vi "App_Main.vi"() -> ()   [LabVIEW 2012]
uses:
  SupportVi/LineStateLamp.ctl
  Fun/Dev/SupportVi/DevState.ctl
  Fun/Dev/DevControl.lvclass
  SupportVi/SystemState.ctl
  Fun/Http/HttpClient.lvclass
  SupportVi/Dev_State_Color.ctl
  <vilib>/Utility/miscctls.llb/LVRowAndColumnTypeDef.ctl
  Fun/Dev/SupportVi/LampState.ctl
  Libs/Ini/ProcessMode.ctl
  <vilib>/Utility/miscctls.llb/LVRowAndColumnUnsignedTypeDef.ctl
  Libs/Ini/IniReader&WriterForControl.lvlib
panel:
  out "Fac&FloChkOK?":bool
  out "HttpClient":refnum<class "HttpClient.lvclass">
  out "FloorCode":string
  out "FactoryCode":string
  out "有變化的部分":string
  in  "Ïµ½y î‘B":T1=enum."Quit"
  out "ˆó¾¯Æ÷":refnum<class "DevControl.lvclass">
  out "需要掃描的":T3(array[cluster])
  out "所有的":cluster{"Addr":u8, "Enable?":bool}[](array[cluster])
  out "History":path
  out "Port":refnum<visa-resource-name>
  out "ConfigFile":path
  out "DataUpload":bool
  out "ReadDelay":i32
  out "SerialRetry":i32
  out "LampBaudRate":i32
  out "BaudRate":i32
  in  "VerifyTimes":i32
  out "DataUrl":string
  out "Model":string
  out "Line":string
  out "Floor":string
  out "Factory":string
  out "RootPath":path
  in  "運行信息":string
  out "版本信息":string
  out "LineState":T4
  out "No-Reply":u32(colorbox)
  out "Abnormal":u32(colorbox)
  in  "ESDShower":string[][](table)
  out "Normal":u32(colorbox)
  in  "Stop":bool
  in  "Start":bool
  # "ESD Monitor System"
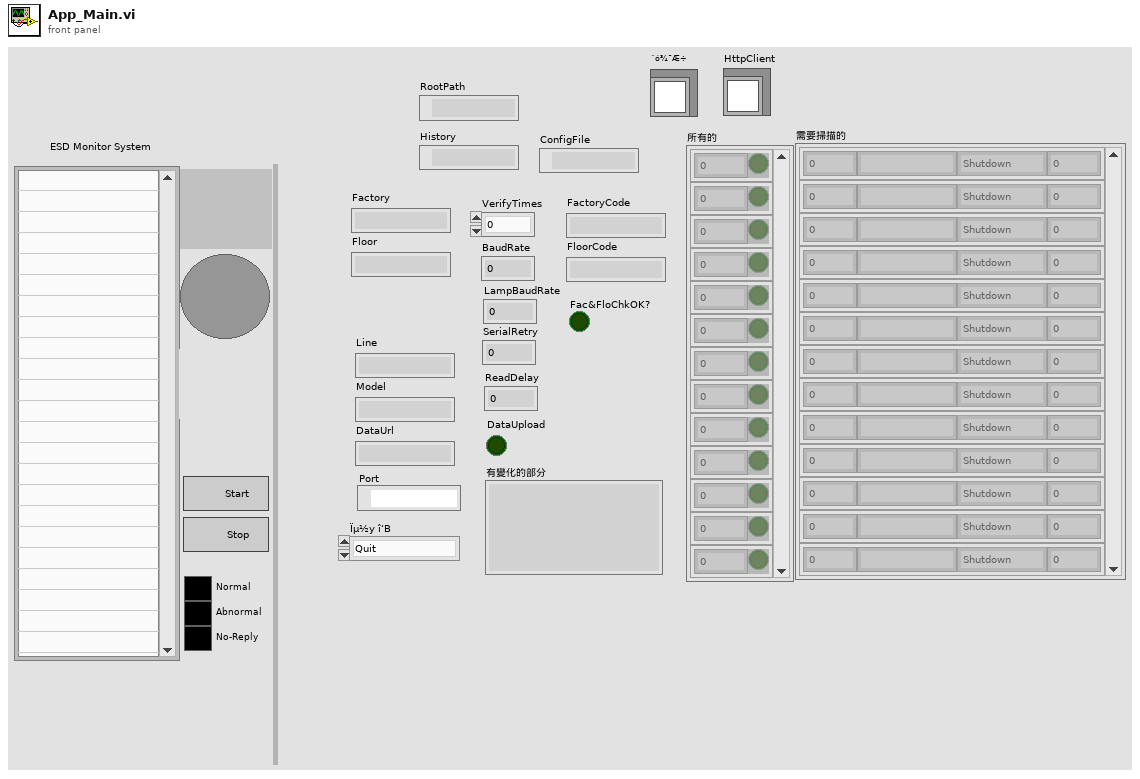
[diagram p1: front panel]
types:
  T1 = typedef "SystemState.ctl" = enum16{"Pause", "Quit", "Error", "Stopping", "Starting", "Init", "Scan", "Menu", "ReadConf", "Idle"}
  T2 = typedef "DevControl.lvclass/DevState.ctl" = enum16{"Shutdown", "PASS", "FAIL", "Idle", "Noresponse"}
  T3 = cluster{"Addr":u8, "name":string, "State":T2, "Retry":i32}[]
  T4 = typedef "LineStateLamp.ctl" = bool
  T5 = typedef "Dev_State_Color.ctl" = u32
  T6 = typedef "IniReader&WriterForControl.lvlib/ProcessMode.ctl" = enum16{"读", "写"}
  T7 = enum8{"Enabled", "Disabled", "Disabled and Grayed Out"}
  T8 = typedef "LVRowAndColumnUnsignedTypeDef.ctl" = cluster{"Row":u32, "Column":u32}
  T9 = cluster{"Addr":i32, "name":string, "State":T2, "Retry":i32}[]
  T10 = typedef "LVRowAndColumnTypeDef.ctl" = cluster{"Row":i32, "Column":i32}
  T11 = typedef "DevControl.lvclass/LampState.ctl" = enum16{"üS+·äøQÆ÷", "¼t+·äøQÆ÷", "·äøQÆ÷", "È«œç", "全亮", "üS", "¾G", "¼t"}
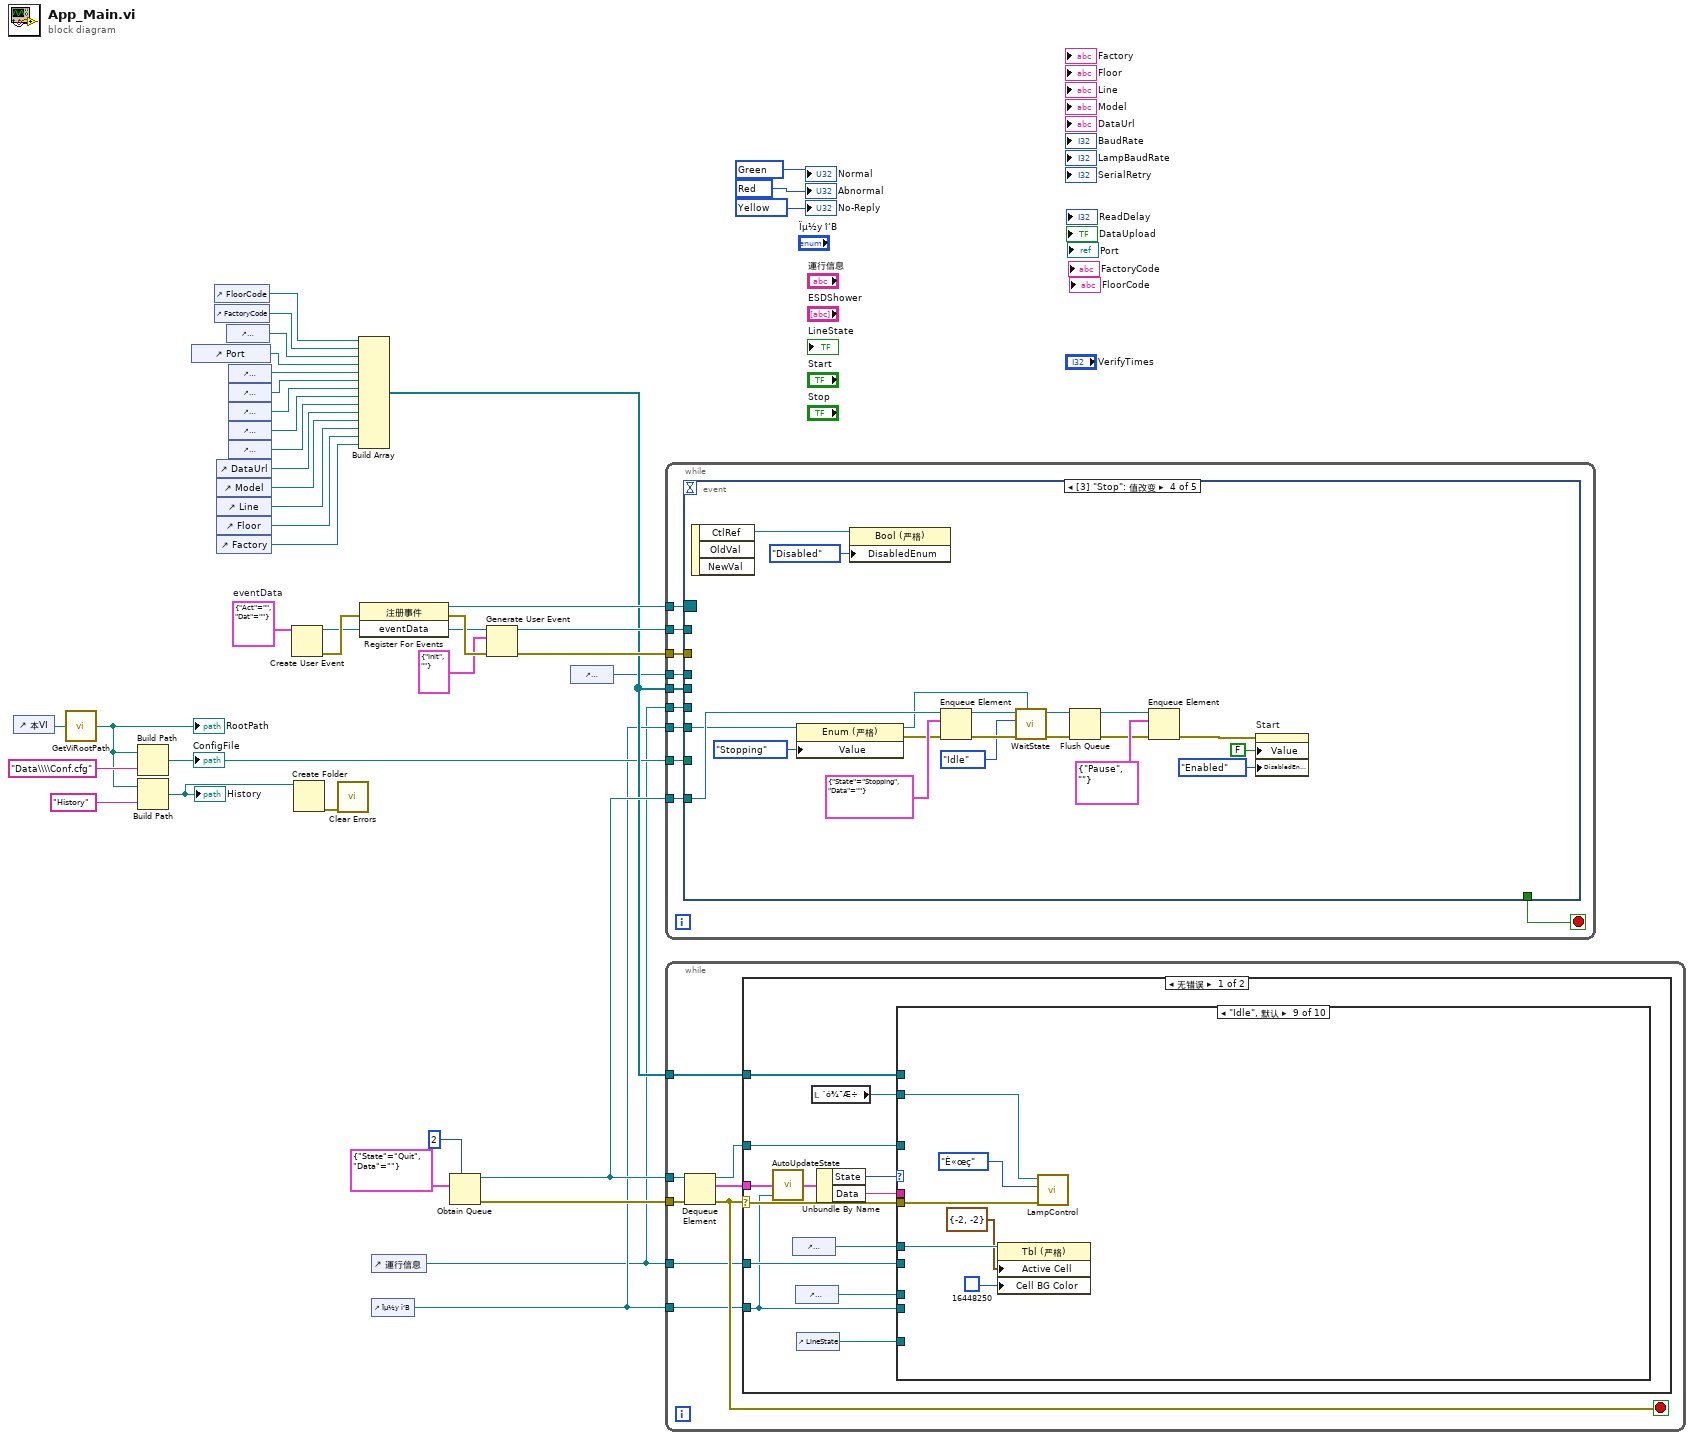
[diagram p0: block diagram]
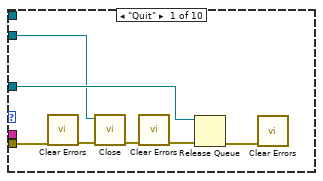
[diagram p2: hidden frame]
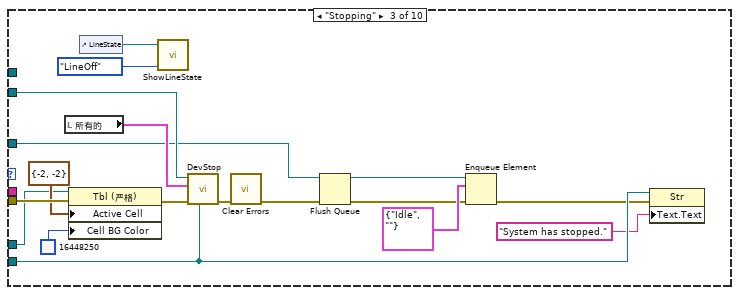
[diagram p4: hidden frame]
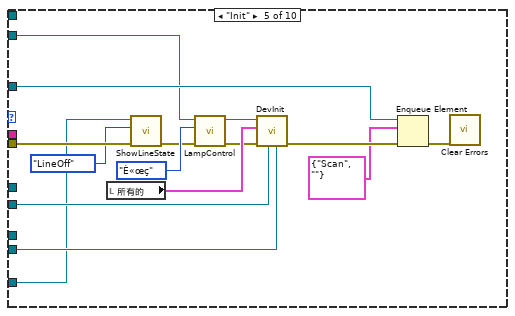
[diagram p6: hidden frame]
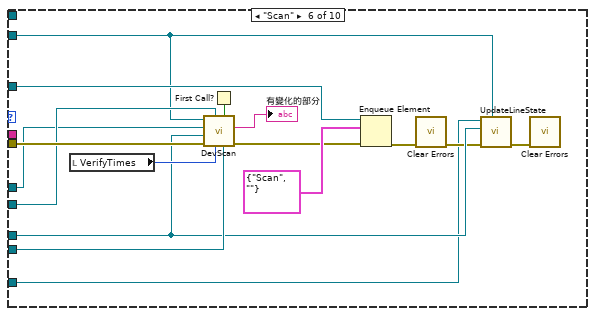
[diagram p7: hidden frame]
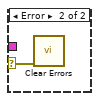
[diagram p11: hidden frame]
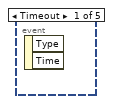
[diagram p12: hidden frame]
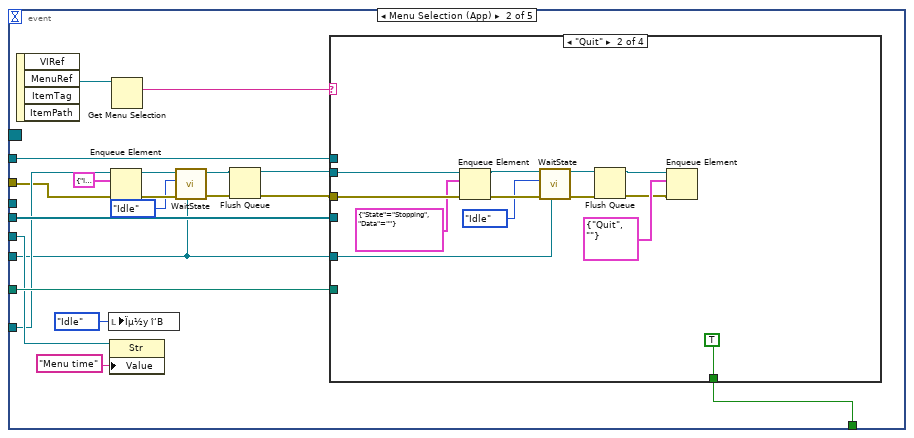
[diagram p13: hidden frame]
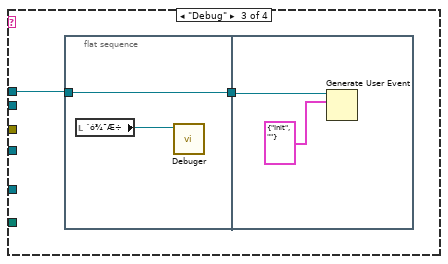
[diagram p15: hidden frame]
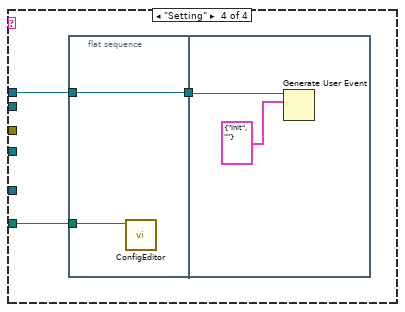
[diagram p16: hidden frame]
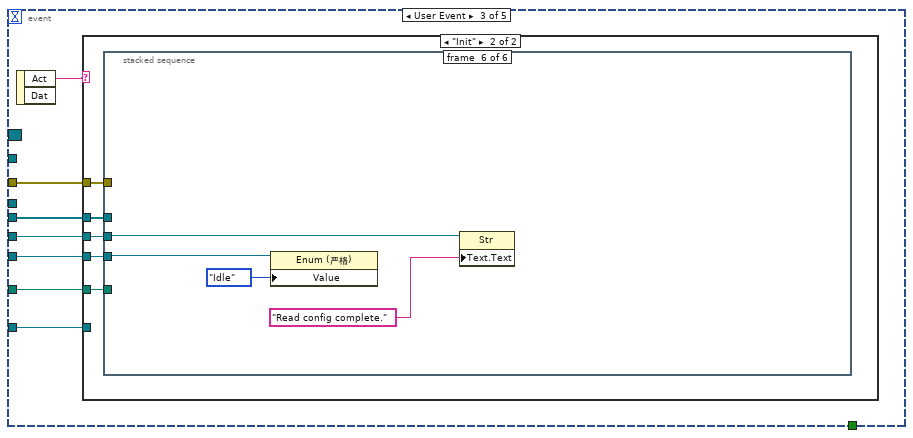
[diagram p17: hidden frame]
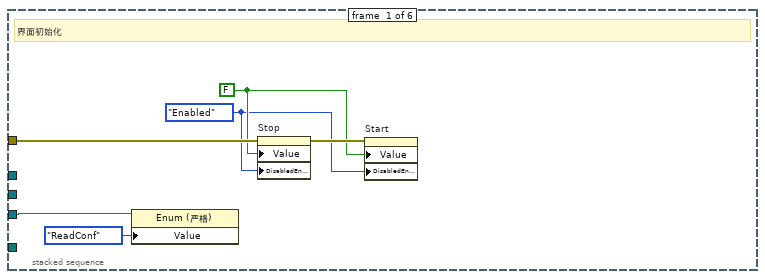
[diagram p19: hidden frame]
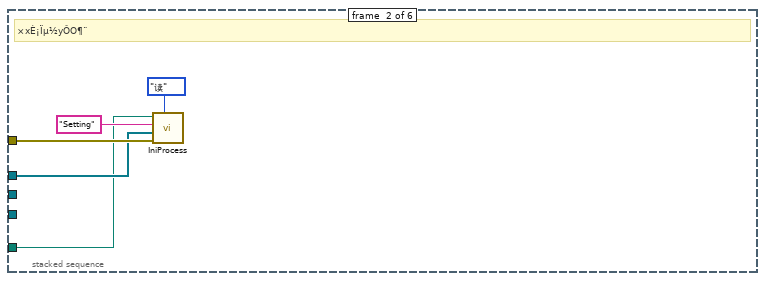
[diagram p20: hidden frame]
diagram:
  w32 = cluster{"Act":string, "Dat":string} {"Act"="", "Dat"=""}  # eventData
  w38 = T5 16772209 items=["Yellow"=16772209, "Red"=16711680, "Green"=6618880] ("DevState_Color")
  w39 = T5 16711680 items=["Yellow"=16772209, "Red"=16711680, "Green"=6618880] ("DevState_Color")
  w40 = T5 6618880 items=["Yellow"=16772209, "Red"=16711680, "Green"=6618880] ("DevState_Color")
  n1 = control-ref of="本VI"() -> (w37:refnum<vi>)
  n2 = call "GetViRootPath.vi"("VI引用句柄"=w37) -> ("RootPath"=w12:path)
  "RootPath" <- w12
  n3 = Build Path(base path=w12, name or relative path="Data\\\\Conf.cfg" ("名称或相对路径")) -> (appended path=w7:path)
  "ConfigFile" <- w7
  n4 = Build Path(base path=w12, name or relative path="History" ("名称或相对路径")) -> (appended path=w10:path)
  "History" <- w10
  n5 = control-ref of="Port"() -> (w14:refnum<vi>)
  n6 = control-ref of="FloorCode"() -> (w2:refnum<vi>)
  n7 = control-ref of="FactoryCode"() -> (w3:refnum<vi>)
  n8 = control-ref of="DataUrl"() -> (w20:refnum<vi>)
  n9 = control-ref of="Model"() -> (w19:refnum<vi>)
  n10 = control-ref of="Line"() -> (w18:refnum<vi>)
  n11 = control-ref of="Floor"() -> (w17:refnum<vi>)
  n12 = control-ref of="Factory"() -> (w16:refnum<vi>)
  n13 = control-ref of="VerifyTimes"() -> (w13:refnum<vi>)
  n14 = control-ref of="DataUpload"() -> (w25:refnum<vi>)
  n15 = control-ref of="ReadDelay"() -> (w24:refnum<vi>)
  n16 = control-ref of="SerialRetry"() -> (w23:refnum<vi>)
  n17 = control-ref of="LampBaudRate"() -> (w22:refnum<vi>)
  n18 = control-ref of="BaudRate"() -> (w21:refnum<vi>)
  n19 = Create User Event(user event datatype=w32) -> (user event=w29:refnum<user-event>, error out=w31:errorcluster)  [unwired: 1 in]
  n20 = Create Folder(path (use dialog)=w10) -> (error out=w8:errorcluster)  [unwired: 2 in, 2 out]
  n21 = call <vilib>:"Clear Errors.vi"("error in (no error)"=w8) -> ()  [unwired: 6 in, 1 out]
  n22 = Build Array(w2, w3, w13, w14, w25, w24, w23, w22, w21, w20, w19, w18, w17, w16) -> (w9:refnum<vi>[])
  n23 = register-events(error in=w31, w29) -> (reference out=w33:refnum<event-registration>, error out=w30:errorcluster)  [unwired: 1 in]
  n24 = control-ref of="運行信息"() -> (w5:refnum<vi>)
  n25 = control-ref of="Ïµ½y î‘B"() -> (w6:refnum<vi>)
  n26 = Obtain Queue(max queue size (-1, unlimited)=2 ("队列最大值（-1，无限）"), element data type=cluster{"State":T1, "Data":string} {"State"=enum."Quit", "Data"=""}) -> (queue out=w34:refnum<queue>, error out=w36:errorcluster)  [unwired: 3 in, 1 out]
  n27 = Generate User Event(user event=w29, event data cluster=cluster{"Act":string, "Dat":string} {"Act"="Init", "Dat"=""} ("事件数据"), error in=w30) -> (user event out=w27:refnum<user-event>, error out=w26:errorcluster)
  n28 = control-ref of="ESDShower"() -> (w4:refnum<vi>)
  n29 = while {
    tunnel: w34 -> [w49]
    tunnel: w33 -> [w48]
    tunnel: w27 -> [w47]
    tunnel: w26 -> [w46]
    tunnel: w9 -> [w45]
    tunnel: w7 -> [w44]
    tunnel: w6 -> [w43]
    tunnel: w5 -> [w42]
    tunnel: w4 -> [w41]
    stop <- w50 stop-if-true
    n30 = event shown="[3] \"Stop\": 值改变" {
      selector: w48 -> [_ _ _ _ _]
      dyn-events: _ -> [_ _ _ _ _]
      timeout: _ -> [_ _ _ _ _]
      tunnel: [_ w67 _ _ w191] -> w50
      tunnel: w49 -> [_ w60 w100 w180 w192]
      tunnel: w47 -> [_ w63 _ _ _]
      tunnel: w46 -> [_ w59 w99 _ w184]
      tunnel: w45 -> [_ w65 w98 _ _]
      tunnel: w44 -> [_ w64 w97 _ _]
      tunnel: w43 -> [_ w57 w96 w178 _]
      tunnel: w42 -> [_ w62 w95 _ _]
      tunnel: w41 -> [_ _ _ _ w188]
      event Timeout {
        n31 = event-data() -> ()  [unwired: 1 in, 2 out]
      }
      event Menu Selection (App) {
        n32 = event-data() -> ("MenuRef"=w69:refnum<k9>)  [unwired: 1 in, 3 out]
        n33 = local write "Ïµ½y î‘B"(SystemState."Idle" ("Ïµ½y î‘B")) -> ()
        n34 = property class="Str"(reference=w62, "Value"="Menu time" ("值")) -> ()  [unwired: 1 in, 2 out]
        n35 = Enqueue Element(queue=w60, element=cluster{"State":T1, "Data":string} {"State"=enum."Idle", "Data"=""} ("元素"), error in (no error)=w59) -> (queue out=w53:refnum<queue>, error out=w58:errorcluster)  [unwired: 1 in, 1 out]
        n36 = Get Menu Selection(0:w69) -> (6:w68:string)  [unwired: 3 in, 4 out]
        n37 = call "WaitState.vi"("Enum输入"=w57, "错误输入（无错误）"=w58, "™z²é î‘B"=SystemState."Idle") -> ("错误输出"=w55:errorcluster)  [unwired: 8 in]
        n38 = Flush Queue(queue=w53, error in (no error)=w55) -> (queue out=w52:refnum<queue>, error out=w54:errorcluster)  [unwired: 1 out]
        n39 = case shown="\"Quit\"" w68 {
          tunnel: [_ TRUE _ _] -> w67
          tunnel: w54 -> [_ w78 _ _]
          tunnel: w65 -> [_ _ _ _]
          tunnel: w64 -> [_ _ _ w90]
          tunnel: w52 -> [_ w79 _ _]
          tunnel: w63 -> [_ _ w82 w89]
          tunnel: w57 -> [_ w75 _ _]
          frame "假", Default {
          }
          frame "Quit" {
            n40 = Enqueue Element(queue=w79, element=cluster{"State":T1, "Data":string} {"State"=enum."Stopping", "Data"=""} ("元素"), error in (no error)=w78) -> (queue out=w72:refnum<queue>, error out=w76:errorcluster)  [unwired: 1 in, 1 out]
            n41 = call "WaitState.vi"("Enum输入"=w75, "错误输入（无错误）"=w76, "™z²é î‘B"=SystemState."Idle") -> ("错误输出"=w73:errorcluster)  [unwired: 8 in]
            n42 = Flush Queue(queue=w72, error in (no error)=w73) -> (queue out=w70:refnum<queue>, error out=w71:errorcluster)  [unwired: 1 out]
            n43 = Enqueue Element(queue=w70, element=cluster{"State":T1, "Data":string} {"State"=enum."Quit", "Data"=""} ("元素"), error in (no error)=w71) -> ()  [unwired: 1 in, 3 out]
          }
          frame "Debug" {
            n44 = flat-sequence {
              tunnel: w82 -> [w85]
              tunnel: [w85] -> w83
              tunnel: w83 -> [w87]
              frame #0 {
                n45 = local read "ˆó¾¯Æ÷"() -> (w84:refnum<class "DevControl.lvclass">)
                n46 = call "Debuger.vi"("DevControl输入"=w84) -> ()  [unwired: 11 in]
              }
              frame #1 {
                n47 = Generate User Event(user event=w87, event data cluster=cluster{"Act":string, "Dat":string} {"Act"="Init", "Dat"=""} ("事件数据")) -> ()  [unwired: 1 in, 2 out]
              }
            }
          }
          frame "Setting" {
            n48 = flat-sequence {
              tunnel: w90 -> [w92]
              tunnel: w89 -> [w91]
              tunnel: [w91] -> w88
              tunnel: w88 -> [w94]
              frame #0 {
                n49 = call "ConfigEditor.vi"("ConfigFile"=w92) -> ()  [unwired: 11 in]
              }
              frame #1 {
                n50 = Generate User Event(user event=w94, event data cluster=cluster{"Act":string, "Dat":string} {"Act"="Init", "Dat"=""} ("事件数据")) -> ()  [unwired: 1 in, 2 out]
              }
            }
          }
        }
      }
      event User Event {
        n51 = event-data() -> ("Act"=w101:string)  [unwired: 1 in, 1 out]
        n52 = case shown="\"Init\"" w101 {
          tunnel: w100 -> [_ _]
          tunnel: w99 -> [_ w106]
          tunnel: w98 -> [_ w105]
          tunnel: w97 -> [_ w104]
          tunnel: w96 -> [_ w103]
          tunnel: w95 -> [_ w102]
          frame "假", Default {
          }
          frame "Init" {
            n53 = stacked-sequence {
              tunnel: w106 -> [w110 w115 w118 w136 w138 _]
              tunnel: w105 -> [_ w114 _ _ _ _]
              tunnel: w104 -> [_ w113 w120 _ _ _]
              tunnel: w103 -> [w112 _ _ _ _ w162]
              tunnel: w102 -> [_ _ _ _ _ w160]
              frame #0 {
                w107 = T7."Enabled" ("禁用")
                w108 = FALSE ("Stop")
                # "界面初始化"
                n54 = property class="Enum (严格)"(reference=w112, "Value"=SystemState."ReadConf" ("值")) -> ()  [unwired: 1 in, 2 out]
                n55 = property on="Stop" class="Bool (严格)"(error in=w110, "Value"=w108, "DisabledEnum"=w107) -> (error out=w109:errorcluster)  [unwired: 1 in, 1 out]
                n56 = property on="Start" class="Bool (严格)"(error in=w109, "Value"=w108, "DisabledEnum"=w107) -> ()  [unwired: 1 in, 2 out]
              }
              frame #1 {
                # "×xÈ¡Ïµ½yÔO¶¨"
                n57 = call "IniProcess.vi"("操作模式"=ProcessMode."读", "error in (no error)"=w115, "Ctls"=w114, "section"="Setting", "configuration file path"=w113) -> ()  [unwired: 5 in, 2 out]
              }
              frame #2 {
                # "×xÈ¡¾€ówÔO¶¨"
                n58 = local read "Model"() -> (w119:string)
                n59 = call "GetDevInfo.vi"("错误输入（无错误）"=w118, "Model"=w119, "ConfigFile"=w120) -> ("error out"=w121:errorcluster, "需要掃描的"=→"需要掃描的":T9, "所有的"=→"所有的":cluster{i32, bool}[])  [unwired: 6 in]
                n60 = stacked-sequence {
                  tunnel: w121 -> [_]
                  frame #0 {
                    n61 = local read "Factory"() -> (w127:string)
                    n62 = local read "Model"() -> (w124:string)
                    n63 = local read "Floor"() -> (w126:string)
                    n64 = local read "Line"() -> (w125:string)
                    n65 = Format Into String(format string=" Version: %s\nFactory: %s\n    Floor: %s\n      Line: %s\nModel: \n%s", "3.00" ("输入 1"), w127, w126, w125, w124) -> (resulting string=→"版本信息":string)  [unwired: 2 in, 1 out]
                  }
                }
              }
              frame #3 {
                # "初始化顯示列表"
                n66 = control-ref of="需要掃描的"() -> (w131:refnum<vi>)
                n67 = control-ref of="ESDShower"() -> (w135:refnum<vi>)
                n68 = control-ref of="LineState"() -> (w133:refnum<vi>)
                n69 = call "InitShower.vi"("error in (no error)"=w136, "DevInfo"=w131, "ï@Ê¾¿ò"=w135) -> ("error out"=w134:errorcluster)  [unwired: 8 in]
                n70 = call "ShowLineState.vi"("错误输入（无错误）"=w134, "LineState"=enum16{"LineOff", "FAIL", "PASS"}."LineOff", "¾€ów î‘BÒýÓÃ"=w133) -> ()  [unwired: 8 in, 1 out]
              }
              frame #4 {
                # "½¨Á¢Http, «@È¡S^ÇÓÐÅÏ¢"
                n71 = local read "DataUpload"() -> (w137:bool)
                n72 = case shown="真" w137 {
                  tunnel: w138 -> [_ w156]
                  frame False {
                  }
                  frame True {
                    n73 = local read "DataUrl"() -> (w152:string)
                    n74 = local read "FactoryCode"() -> (w145:string)
                    n75 = local read "FloorCode"() -> (w146:string)
                    n76 = call-dynamic "Init.vi"("error in (no error)"=w156, "Url"=w152, "HttpClient 输入"=refnum<class "HttpClient.lvclass"> refnum) -> ("error out"=w154:errorcluster, "HttpClient 输出"=w153:refnum<class "HttpClient.lvclass">)  [unwired: 7 in]
                    n77 = call-dynamic "GetFactory&Floor.vi"("error in (no error)"=w154, "模式"=enum16{"˜ÇŒÓ", "S^"}."˜ÇŒÓ", "HttpClient 输入"=w153) -> ("error out"=w150:errorcluster, "Data"=w149:string[][], "HttpClient 输出"=w151:refnum<class "HttpClient.lvclass">)  [unwired: 6 in]
                    n78 = call-dynamic "GetFactory&Floor.vi"("error in (no error)"=w150, "模式"=enum16{"˜ÇŒÓ", "S^"}."S^", "HttpClient 输入"=w151) -> ("error out"=w140:errorcluster, "Data"=w144:string[][], "HttpClient 输出"=→"HttpClient":refnum<class "HttpClient.lvclass">)  [unwired: 6 in]
                    n79 = call <vilib>:"Clear Errors.vi"("error in (no error)"=w140) -> ()  [unwired: 6 in, 1 out]
                    n80 = call "ChkElekExist.vi"("Data"=w144, "Floor"=w145) -> ("布尔"=w143:bool)
                    n81 = call "ChkElekExist.vi"("Data"=w149, "Floor"=w146) -> ("布尔"=w142:bool)
                    n82 = Or(x=w143, y=w142) -> (x .or. y?=w139:bool)
                    "Fac&FloChkOK?" <- w139
                    n83 = case shown="真" w139 {
                      frame False {
                        n84 = One Button Dialog(message="Factory code or floor code check fail, \nCheck that it is correct. \nOr make sure  network is OK." ("消息"), button name ("OK")="OK" ("按钮名称（“确定”）")) -> ()  [unwired: 1 out]
                      }
                      frame True {
                      }
                    }
                  }
                }
              }
              frame #5 {
                n85 = property class="Enum (严格)"(reference=w162, "Value"=SystemState."Idle" ("值")) -> ()  [unwired: 1 in, 2 out]
                n86 = property class="Str"(reference=w160, "Text.Text"="Read config complete." ("文本.文本")) -> ()  [unwired: 1 in, 2 out]
              }
            }
          }
        }
      }
      event "Stop": Value Change {
        n87 = event-data() -> ("CtlRef"=w174:refnum<vi>)  [unwired: 1 in, 2 out]
        n88 = property class="Enum (严格)"(reference=w178, "Value"=SystemState."Stopping" ("值")) -> (reference out=w168:refnum<vi>, error out=w172:errorcluster)  [unwired: 1 in]
        n89 = property class="Bool (严格)"(reference=w174, "DisabledEnum"=T7."Disabled" ("禁用")) -> ()  [unwired: 1 in, 2 out]
        n90 = Enqueue Element(queue=w180, element=cluster{"State":T1, "Data":string} {"State"=enum."Stopping", "Data"=""} ("元素"), error in (no error)=w172) -> (queue out=w164:refnum<queue>, error out=w171:errorcluster)  [unwired: 1 in, 1 out]
        n91 = call "WaitState.vi"("Enum输入"=w168, "错误输入（无错误）"=w171, "™z²é î‘B"=SystemState."Idle") -> ("错误输出"=w166:errorcluster)  [unwired: 8 in]
        n92 = Flush Queue(queue=w164, error in (no error)=w166) -> (queue out=w163:refnum<queue>, error out=w165:errorcluster)  [unwired: 1 out]
        n93 = Enqueue Element(queue=w163, element=cluster{"State":T1, "Data":string} {"State"=enum."Pause", "Data"=""} ("元素"), error in (no error)=w165) -> (error out=w169:errorcluster)  [unwired: 1 in, 2 out]
        n94 = property on="Start" class="Bool (严格)"(error in=w169, "Value"=FALSE ("Stop"), "DisabledEnum"=T7."Enabled" ("禁用")) -> ()  [unwired: 1 in, 2 out]
      }
      event "Start": Value Change {
        n95 = event-data() -> ("CtlRef"=w182:refnum<vi>)  [unwired: 1 in, 2 out]
        n96 = property class="Tbl (严格)"(reference=w188, error in=w184, "Index Values"=T8 {"Row"=0, "Column"=0} ("索引值")) -> (error out=w183:errorcluster)  [unwired: 1 out]
        n97 = property on="Stop" class="Bool (严格)"("Value"=FALSE ("Stop"), "DisabledEnum"=T7."Enabled" ("禁用")) -> ()  [unwired: 2 in, 2 out]
        n98 = property class="Bool (严格)"(reference=w182, "DisabledEnum"=T7."Disabled" ("禁用")) -> ()  [unwired: 1 in, 2 out]
        n99 = local read "ReadDelay"() -> (w194:i32)
        n100 = local read "SerialRetry"() -> (w189:i32)
        n101 = local read "BaudRate"() -> (w195:i32)
        n102 = local read "Port"() -> (w196:refnum<visa-resource-name>)
        n103 = call-dynamic "Init.vi"("DevControl 输入"=refnum<class "DevControl.lvclass"> refnum, "控制端口"=w196, "波特率"=w195, "ReadDelay"=w194, "error in (no error)"=w183, "Retry"=w189) -> ("DevControl 输出"=→"ˆó¾¯Æ÷":refnum<class "DevControl.lvclass">, "error out"=w193:errorcluster)  [unwired: 8 in]
        n104 = case shown="错误" w193 {
          selector: w193 -> [_ w204]
          tunnel: w192 -> [w199 w201]
          tunnel: [_ w200] -> w191
          frame No Error {
            n105 = Enqueue Element(queue=w199, element=cluster{"State":T1, "Data":string} {"State"=enum."Init", "Data"=""} ("元素")) -> ()  [unwired: 2 in, 3 out]
          }
          frame Error {
            n106 = call <vilib>:"Clear Errors.vi"("error in (no error)"=w204) -> ()  [unwired: 6 in, 1 out]
            n107 = One Button Dialog(message="Port open failed. \nPlease check  the port number is correct. \nSystem will be stop." ("消息"), button name ("OK")="OK" ("按钮名称（“确定”）")) -> (true=w200:bool)
            n108 = stacked-sequence {
              tunnel: w201 -> [w205]
              tunnel: w200 -> [_]
              frame #0 {
                n109 = Release Queue(queue=w205) -> ()  [unwired: 2 in, 3 out]
              }
            }
          }
        }
      }
    }
  }
  n110 = while {
    tunnel: w34 -> [w213]
    tunnel: w36 -> [w212]
    tunnel: w9 -> [w208]
    tunnel: w5 -> [w207]
    tunnel: w6 -> [w206]
    stop <- w209 stop-if-true
    n111 = Dequeue Element(queue=w213, error in (no error)=w212) -> (queue out=w210:refnum<queue>, element=w211:cluster{"State":T1, "Data":string}, error out=w209:errorcluster)  [unwired: 1 in, 1 out]
    n112 = case shown="无错误" w209 {
      selector: w209 -> [w222 w289]
      tunnel: w211 -> [w220 _]
      tunnel: w210 -> [w224 _]
      tunnel: w208 -> [w223 _]
      tunnel: w207 -> [w221 _]
      tunnel: w206 -> [w218 _]
      frame No Error {
        n113 = call "AutoUpdateState.vi"("Ïµ½y î‘B"=w218, "ê ÁÐ”µ“þ"=w220) -> ("ê ÁÐ”µ“þ"=w219:cluster{"State":T1, "Data":string})  [unwired: 3 in]
        n114 = control-ref of="ESDShower"() -> (w216:refnum<vi>)
        n115 = control-ref of="需要掃描的"() -> (w215:refnum<vi>)
        n116 = control-ref of="LineState"() -> (w214:refnum<vi>)
        n117 = local read "ˆó¾¯Æ÷"() -> (w217:refnum<class "DevControl.lvclass">)
        n118 = Unbundle By Name(w219) -> ("State"=w226:T1, "Data"=w225:string)
        n119 = case shown="\"Idle\", 默认" w226 {
          tunnel: w225 -> [_ _ _ _ _ _ _ _ _ _]
          tunnel: w224 -> [w233 _ w236 _ w262 w278 _ _ _ _]
          tunnel: w223 -> [_ _ _ _ _ _ _ _ _ _]
          tunnel: w222 -> [w231 _ w247 _ w255 w282 _ _ w285 _]
          tunnel: w221 -> [_ _ w249 _ w265 w276 _ _ _ _]
          tunnel: w218 -> [_ _ _ _ w264 w280 _ _ _ _]
          tunnel: w217 -> [w227 _ w240 _ w257 w268 _ _ w284 _]
          tunnel: w216 -> [_ _ w243 _ _ w273 _ _ w288 _]
          tunnel: w215 -> [_ _ _ _ _ w272 _ _ _ _]
          tunnel: w214 -> [_ _ _ _ w253 w269 _ _ _ _]
          frame "Quit" {
            n120 = call <vilib>:"Clear Errors.vi"("error in (no error)"=w231) -> ("error out"=w230:errorcluster)  [unwired: 6 in]
            n121 = call-dynamic "Close.vi"("error in (no error)"=w230, "DevControl 输入"=w227) -> ("error out"=w229:errorcluster)  [unwired: 8 in, 1 out]
            n122 = call <vilib>:"Clear Errors.vi"("error in (no error)"=w229) -> ("error out"=w228:errorcluster)  [unwired: 6 in]
            n123 = Release Queue(queue=w233, error in (no error)=w228) -> (error out=w232:errorcluster)  [unwired: 1 in, 2 out]
            n124 = call <vilib>:"Clear Errors.vi"("error in (no error)"=w232) -> ()  [unwired: 6 in, 1 out]
          }
          frame "Error" {
          }
          frame "Stopping" {
            n125 = local read "所有的"() -> (w239:cluster{"Addr":u8, "Enable?":bool}[])
            n126 = property class="Tbl (严格)"(reference=w243, error in=w247, "Active Cell"=T10 {"Row"=-2, "Column"=-2} ("活动单元格:活动单元格"), "Cell BG Color"=u32 16448250) -> (error out=w246:errorcluster)  [unwired: 1 out]
            n127 = control-ref of="LineState"() -> (w242:refnum<vi>)
            n128 = call "ShowLineState.vi"("LineState"=enum16{"LineOff", "FAIL", "PASS"}."LineOff", "¾€ów î‘BÒýÓÃ"=w242) -> ()  [unwired: 9 in, 1 out]
            n129 = call "DevStop.vi"("運行信息"=w249, "错误输入（无错误）"=w246, "所有的"=w239, "DevControl输入"=w240) -> ("error out"=w251:errorcluster)  [unwired: 7 in]
            n130 = call <vilib>:"Clear Errors.vi"("error in (no error)"=w251) -> ("error out"=w237:errorcluster)  [unwired: 6 in]
            n131 = Flush Queue(queue=w236, error in (no error)=w237) -> (queue out=w234:refnum<queue>, error out=w235:errorcluster)  [unwired: 1 out]
            n132 = Enqueue Element(queue=w234, element=cluster{"State":T1, "Data":string} {"State"=enum."Idle", "Data"=""} ("元素"), error in (no error)=w235) -> (error out=w238:errorcluster)  [unwired: 1 in, 2 out]
            n133 = property class="Str"(reference=w249, error in=w238, "Text.Text"="System has stopped." ("文本.文本")) -> ()  [unwired: 2 out]
          }
          frame "Starting" {
          }
          frame "Init" {
            n134 = local read "所有的"() -> (w266:cluster{"Addr":u8, "Enable?":bool}[])
            n135 = call "ShowLineState.vi"("错误输入（无错误）"=w255, "LineState"=enum16{"LineOff", "FAIL", "PASS"}."LineOff", "¾€ów î‘BÒýÓÃ"=w253) -> ("错误输出"=w254:errorcluster)  [unwired: 8 in]
            n136 = call-dynamic "LampControl.vi"("error in (no error)"=w254, "ÈýÉ«Ÿô î‘B"=LampState."È«œç", "DevControl 输入"=w257) -> ("error out"=w259:errorcluster, "DevControl 输出"=w258:refnum<class "DevControl.lvclass">)  [unwired: 7 in]
            n137 = call "DevInit.vi"("Ïµ½y î‘B"=w264, "運行信息"=w265, "错误输入（无错误）"=w259, "所有的"=w266, "DevControl输入"=w258) -> ("error out"=w263:errorcluster)  [unwired: 6 in]
            n138 = Enqueue Element(queue=w262, element=cluster{"State":T1, "Data":string} {"State"=enum."Scan", "Data"=""} ("元素"), error in (no error)=w263) -> (error out=w260:errorcluster)  [unwired: 1 in, 2 out]
            n139 = call <vilib>:"Clear Errors.vi"("error in (no error)"=w260) -> ()  [unwired: 6 in, 1 out]
          }
          frame "Scan" {
            n140 = local read "VerifyTimes"() -> (w281:i32)
            n141 = First Call?() -> (First Call?: T/F=w274:bool)
            n142 = call "DevScan.vi"("Ïµ½y î‘B"=w280, "首次調用?"=w274, "VerifyTimes"=w281, "顯示信息"=w276, "错误输入（无错误）"=w282, "需要掃描的"=w272, "ESDShower"=w273, "DevControl输入"=w268) -> ("error out"=w270:errorcluster, "有變化的部分"=→"有變化的部分":string)  [unwired: 2 in]
            n143 = Enqueue Element(queue=w278, element=cluster{"State":T1, "Data":string} {"State"=enum."Scan", "Data"=""} ("元素"), error in (no error)=w270) -> (error out=w275:errorcluster)  [unwired: 1 in, 2 out]
            n144 = call <vilib>:"Clear Errors.vi"("error in (no error)"=w275) -> ("error out"=w271:errorcluster)  [unwired: 6 in]
            n145 = call "UpdateLineState.vi"("DevControl 输入"=w268, "error in (no error)"=w271, "¾€ów”µ“þ"=w272, "¾€ów î‘B"=w269) -> ("error out"=w267:errorcluster)  [unwired: 7 in]
            n146 = call <vilib>:"Clear Errors.vi"("error in (no error)"=w267) -> ()  [unwired: 6 in, 1 out]
          }
          frame "Menu" {
          }
          frame "ReadConf" {
          }
          frame "Idle", Default {
            n147 = property class="Tbl (严格)"(reference=w288, "Active Cell"=T10 {"Row"=-2, "Column"=-2} ("活动单元格:活动单元格"), "Cell BG Color"=u32 16448250) -> ()  [unwired: 1 in, 2 out]
            n148 = call-dynamic "LampControl.vi"("error in (no error)"=w285, "ÈýÉ«Ÿô î‘B"=LampState."È«œç", "DevControl 输入"=w284) -> ()  [unwired: 7 in, 2 out]
          }
          frame "Pause" {
          }
        }
      }
      frame Error {
        n149 = call <vilib>:"Clear Errors.vi"("error in (no error)"=w289) -> ()  [unwired: 6 in, 1 out]
      }
    }
  }
  "Normal" <- w40
  "Abnormal" <- w39
  "No-Reply" <- w38
